vi "Global.vi"() -> ()   [LabVIEW 2016]
panel:
  in  "lastpos":dbl
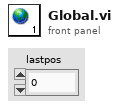
[diagram p1: front panel]
diagram:
